vi "EnableControls.vi"(8 "error in (no error)":errorcluster, 9 "Disabled":T1(ring), 11 "Panel in":refnum<vi>) -> (0 "error out":errorcluster)   [LabVIEW 2023]
panel:
  in  "target class":refnum<vi>
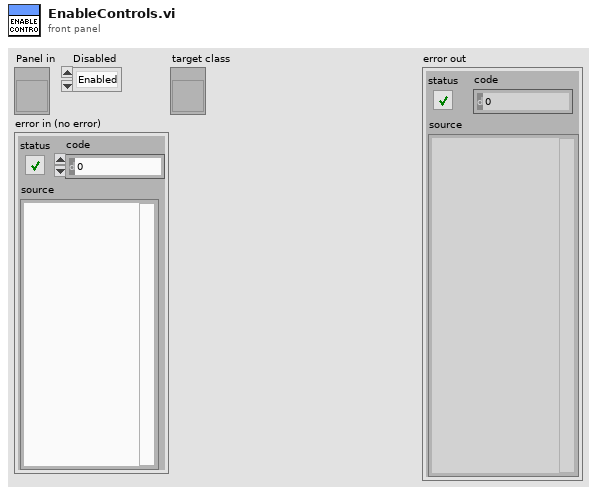
[diagram p1: front panel]
types:
  T1 = enum8{"Enabled", "Disabled", "Disabled and Grayed Out"}
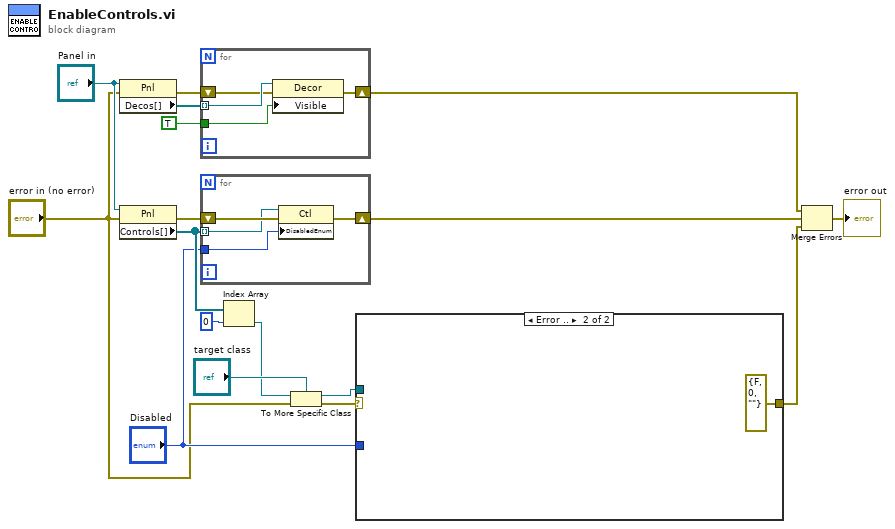
[diagram p0: block diagram]
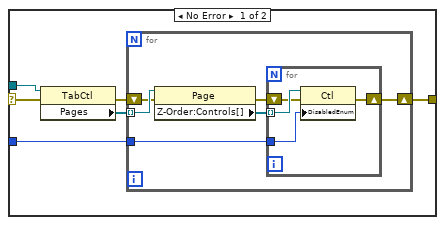
[diagram p2: hidden frame]
diagram:
  n1 = property class="Pnl"(reference="Panel in", error in="error in (no error)") -> (error out=w14:errorcluster, "Decos[]"=w16:refnum<vi>[])  [unwired: 1 out]
  n2 = property class="Pnl"(reference="Panel in", error in="error in (no error)") -> (error out=w13:errorcluster, "Controls[]"=w9:refnum<vi>[])  [unwired: 1 out]
  n3 = for {
    tunnel: w16 -> [w21] mode=indexing
    tunnel: TRUE -> [w20]
    shift-right: [w18] -> w12
    shift-left: w14 -> [w19]
    n4 = property class="Decor"(reference=w21, error in=w19, "Visible"=w20) -> (error out=w18:errorcluster)  [unwired: 1 out]
  }
  n5 = for {
    tunnel: w9 -> [w22] mode=indexing
    tunnel: "Disabled" -> [w25]
    shift-right: [w24] -> w11
    shift-left: w13 -> [w23]
    n6 = property class="Ctl"(reference=w22, error in=w23, "DisabledEnum"=w25) -> (error out=w24:errorcluster)  [unwired: 1 out]
  }
  n7 = Index Array(array=w9, index=0) -> (element=w2:refnum<vi>)
  n8 = To More Specific Class(target class="target class", reference=w2, error in="error in (no error)") -> (specific class reference=w4:refnum<vi>, error out=w1:errorcluster)
  n9 = case shown="Error .." w1 {
    selector: w1 -> [w26 _]
    tunnel: "Disabled" -> [w31 _]
    tunnel: [w30 errorcluster {"status"=FALSE, "code"=0, "source"=""} ("error out")] -> w7
    tunnel: w4 -> [w29 _]
    frame No Error {
      n10 = property class="TabCtl"(reference=w29, error in=w26) -> (error out=w27:errorcluster, "Pages"=w28:refnum<vi>[])  [unwired: 1 out]
      n11 = for {
        tunnel: w28 -> [w37] mode=indexing
        tunnel: w31 -> [w35]
        shift-right: [w34] -> w30
        shift-left: w27 -> [w32]
        n12 = property class="Page"(reference=w37, error in=w32) -> (error out=w33:errorcluster, "Z-Order:Controls[]"=w36:refnum<vi>[])  [unwired: 1 out]
        n13 = for {
          tunnel: w36 -> [w41] mode=indexing
          tunnel: w35 -> [w40]
          shift-right: [w39] -> w34
          shift-left: w33 -> [w38]
          n14 = property class="Ctl"(reference=w41, error in=w38, "DisabledEnum"=w40) -> (error out=w39:errorcluster)  [unwired: 1 out]
        }
      }
    }
    frame Error {
    }
  }
  n15 = Merge Errors(w12, w11, w7) -> (→"error out":errorcluster)
